vi "Delete Heirarchy Rows.vi"(8 "error in (no error)":errorcluster, 11 "Data":T1) -> (0 "error out":errorcluster, 3 "OK":bool)   [LabVIEW 2018]
uses:
  <vilib>/httpClient/LabVIEWHTTPClient.lvlib
  TypeDef/Main - Handle Heirarchy Drag&Drop - Data.ctl
panel:
  out "Bodies":string[](array[string])
  out "Headers":string[](array[string])
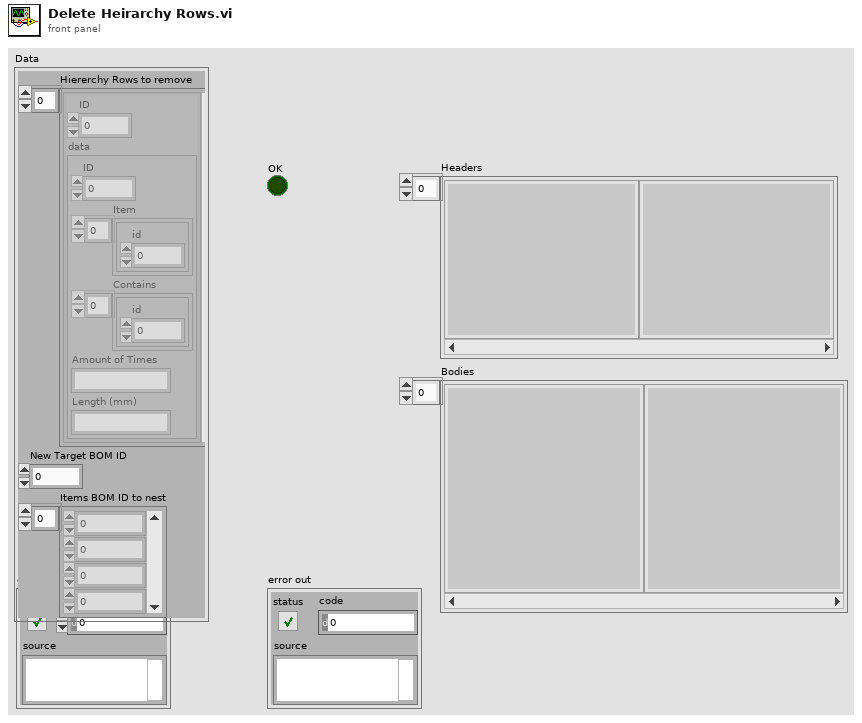
[diagram p1: front panel]
types:
  T1 = typedef "Main - Handle Heirarchy Drag&Drop - Data.ctl" = cluster{"Hiererchy Rows to remove":cluster{"ID":i32, "data":cluster{"ID":i32, "Item":cluster{"id":i32}[], "Contains":cluster{"id":i32}[], "Amount of Times":string, "Length (mm)":string}}[], "New Target BOM ID":i32, "Items BOM ID to nest":i32[]}
  T2 = typedef "LabVIEWHTTPClient.lvlib/ClientHandle.ctl" = refnum<k1>
  T3 = cluster{"ID":i32, "data":cluster{"ID":i32, "Item":cluster{"id":i32}[], "Contains":cluster{"id":i32}[], "Amount of Times":string, "Length (mm)":string}}[]
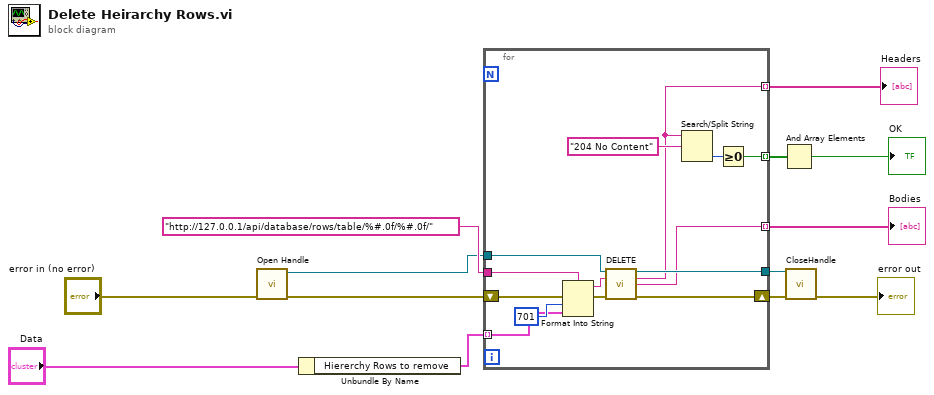
[diagram p0: block diagram]
diagram:
  n1 = call "Open Handle.vi"("error in (no error)"="error in (no error)") -> ("error out"=w10:errorcluster, "Refnum out"=w8:T2)  [unwired: 9 in]
  n2 = Unbundle By Name("Data") -> ("Hiererchy Rows to remove"=w9:T3)
  n3 = for {
    tunnel: "http://127.0.0.1/api/database/rows/table/%#.0f/%#.0f/" ("url") -> [w26]
    shift-right: [w27] -> w7
    shift-left: w10 -> [w24]
    tunnel: w9 -> [w21] mode=indexing
    tunnel: w8 -> [w20]
    tunnel: [w19] -> w5
    tunnel: [w15] -> w4 mode=indexing
    tunnel: [w18] -> w3 mode=indexing
    tunnel: [w14] -> w2 mode=indexing
    n4 = Format Into String(format string=w26, error in=w24, u32 701 ("input 1"), w21) -> (resulting string=w22:string, error out=w23:errorcluster)  [unwired: 1 in]
    n5 = call <vilib>:"DELETE.vi"("client handle"=w20, "url"=w22, "error in (no error)"=w23) -> ("client handle out"=w19:T2, "headers"=w15:string, "body"=w18:string, "error out"=w27:errorcluster)  [unwired: 9 in]
    n6 = Search/Split String(string=w15, search string/char (-)="204 No Content") -> (offset of match=w16:i32)  [unwired: 1 in, 2 out]
    n7 = Greater Or Equal To 0?(x=w16) -> (x >= 0?=w14:bool)
  }
  "Bodies" <- w3
  "Headers" <- w4
  n8 = And Array Elements(Boolean array=w2) -> (logical AND=→"OK":bool)
  n9 = call <vilib>:"CloseHandle.vi"("client handle"=w5, "error in (no error)"=w7) -> ("error out"=→"error out":errorcluster)  [unwired: 13 in]
